vi "XY Graph Compute Convolution Product Event.vi"(6 "Reference Decay":T1, 8 "Error In":errorcluster, 9 "Valid Reference Decay?":bool, 10 "Plot at Coordinates":i32, 11 "Multiplot XY Graph":T2) -> (0 "Error Out":errorcluster, 1 "Message":string, 3 "Plot Name":string)   [LabVIEW 2021, in "XY Graph Add-Ons.lvlib"]
uses:
  XY Graph Add-Ons.lvlib
  XY Graph Refnum.ctl
  XY Plot Data.ctl
  Fits/Fits.lvlib
  Math/Math.lvlib
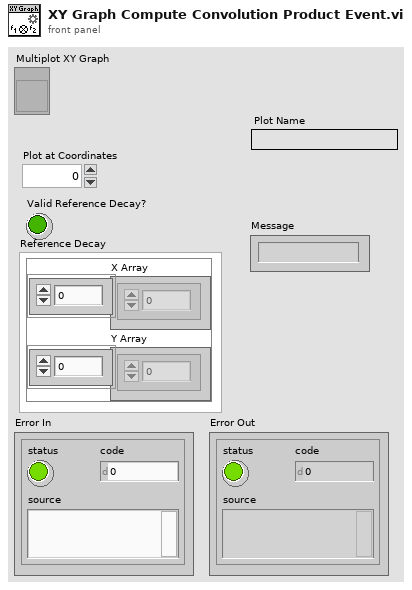
[diagram p1: front panel]
types:
  T1 = typedef "XY Graph Add-Ons.lvlib/XY Plot Data.ctl" = cluster{"X Array":dbl[], "Y Array":dbl[]}
  T2 = typedef "XY Graph Add-Ons.lvlib/XY Graph Refnum.ctl" = refnum<vi>
  T3 = typedef "Graphs.lvlib/Plot Destination.ctl" = enum32{"Plot 1", "Plot 2", "New Plot"}
  T4 = typedef "XY Graph Add-Ons.lvlib/XY Graph Convolution Product Options.ctl" = cluster{"Plot 1":u16, "Plot 2":u16, "Period Type":T5, "Period":dbl[unit], "Time Step":T6, "Step":dbl[unit]}
  T5 = typedef "XY Graph Add-Ons.lvlib/XY Graph Convolution Period Type.ctl" = enum16{"Laser", "Plot 1 Duration", "Plot 2 Duration", "User Defined"}
  T6 = typedef "XY Graph Add-Ons.lvlib/XY Graph Convolution Step Type.ctl" = enum16{"Plot 1 Step", "Plot 2 Step", "User Defined"}
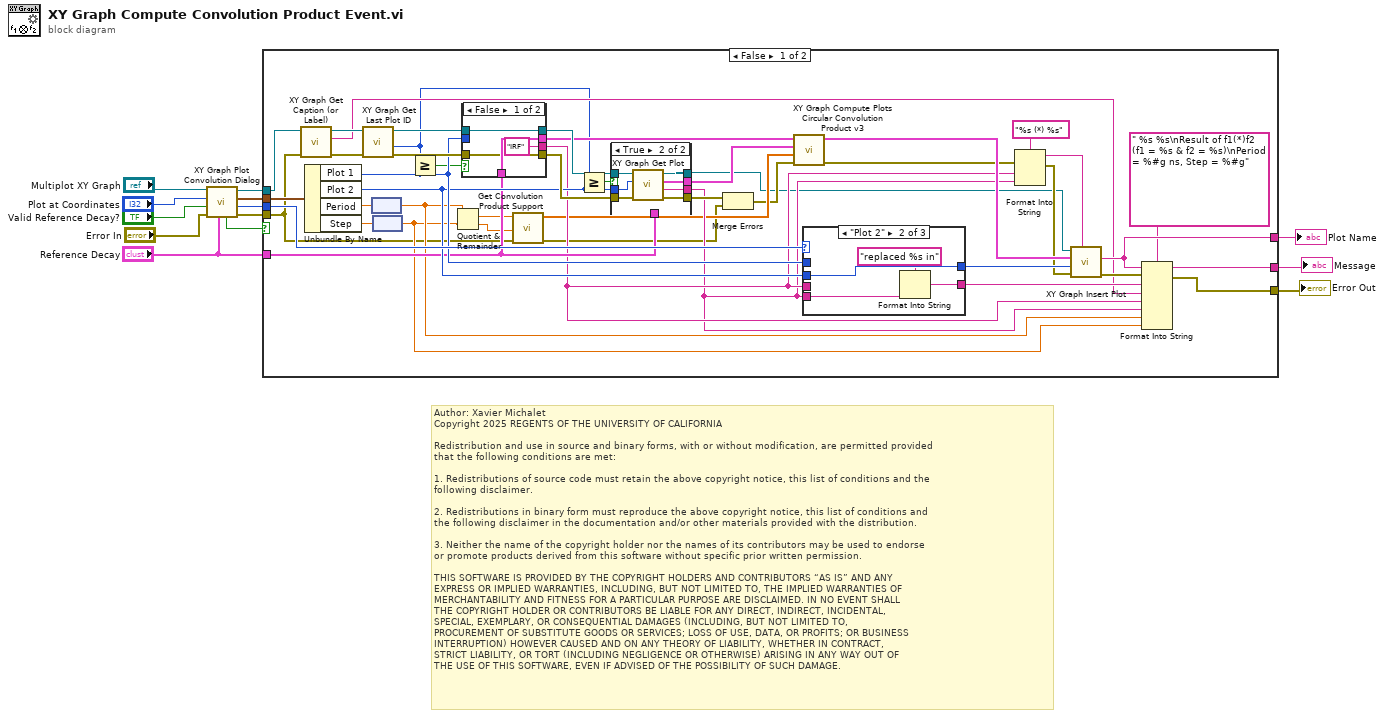
[diagram p0: block diagram]
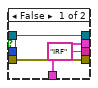
[diagram p2: hidden frame]
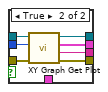
[diagram p3: hidden frame]
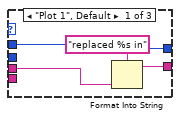
[diagram p4: hidden frame]
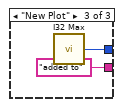
[diagram p5: hidden frame]
diagram:
  # "Author: Xavier Michalet\nCopyright 2025 REGENTS OF THE UNIVERSITY OF CALIFORNIA\n\nRedistribution and use in source and binary forms, with or without modification, are permitted provided\nthat the following conditions are met:\n\n1. Redistributions of source code must retain the above copyright notice, this list of conditions and the\nfollowing disclaimer.\n\n2. Redistributions in binary form must reproduce the above copyright notice, this list of conditions and\nthe following disclaimer in the documentation and/or other materials provided with the distribution.\n\n3. Neither the name of the copyright holder nor the names of its contributors may be used to endorse \nor promote products derived from this software without specific prior written permission.\n\nTHIS SOFTWARE IS PROVIDED BY THE COPYRIGHT HOLDERS AND CONTRIBUTORS “AS IS” AND ANY \nEXPRESS OR IMPLIED WARRANTIES, INCLUDING, BUT NOT LIMITED TO, THE IMPLIED WARRANTIES OF\nMERCHANTABILITY AND FITNESS FOR A PARTICULAR PURPOSE ARE DISCLAIMED. IN NO EVENT SHALL\nTHE COPYRIGHT HOLDER OR CONTRIBUTORS BE LIABLE FOR ANY DIRECT, INDIRECT, INCIDENTAL, \nSPECIAL, EXEMPLARY, OR CONSEQUENTIAL DAMAGES (INCLUDING, BUT NOT LIMITED TO, \nPROCUREMENT OF SUBSTITUTE GOODS OR SERVICES; LOSS OF USE, DATA, OR PROFITS; OR BUSINESS\nINTERRUPTION) HOWEVER CAUSED AND ON ANY THEORY OF LIABILITY, WHETHER IN CONTRACT, \nSTRICT LIABILITY, OR TORT (INCLUDING NEGLIGENCE OR OTHERWISE) ARISING IN ANY WAY OUT OF\nTHE USE OF THIS SOFTWARE, EVEN IF ADVISED OF THE POSSIBILITY OF SUCH DAMAGE."
  n1 = call "XY Graph Plot Convolution Dialog.vi"("Reference Decay"="Reference Decay", "Error In"="Error In", "Valid Reference Decay?"="Valid Reference Decay?", "Plot at Coordinates"="Plot at Coordinates", "XY Graph"="Multiplot XY Graph") -> ("Error Out"=w6:errorcluster, "Plot Destination out"=w4:T3, "Convolution Product Options out"=w3:T4, "XY Graph (dup)"=w2:refnum<vi>, "Cancelled"=w5:bool)  [unwired: 2 in]
  n2 = case shown="False" w5 {
    tunnel: [w56 w89] -> w13
    tunnel: [w55 _] -> w12
    tunnel: [w54 _] -> w11
    tunnel: w6 -> [w17 w89]
    tunnel: w4 -> [w53 _]
    tunnel: w3 -> [w52 _]
    tunnel: w2 -> [w44 _]
    tunnel: "Reference Decay" -> [w28 _]
    frame False {
      n3 = call "XY Graph Get Caption (or Label).vi"("error in (no error)"=w17, "XYGraph in"=w44) -> ("error out"=w34:errorcluster, "Caption (or Label) Text"=w33:string, "XYGraph out"=w35:T2)  [unwired: 7 in]
      n4 = Unbundle By Name(w52) -> ("Plot 1"=w36:u16, "Plot 2"=w31:u16, "Period"=w47:dbl[unit], "Step"=w46:dbl[unit])
      n5 = call "XY Graph Get Last Plot ID.vi"("error in (no error)"=w34, "XYGraph in"=w35) -> ("error out"=w37:errorcluster, "Last Plot ID"=w30:i32, "XYGraph out"=w38:refnum<vi>)  [unwired: 7 in]
      n6 = node(w47) -> (w21:dbl)
      n7 = node(w46) -> (w20:dbl)
      n8 = Greater Or Equal?(x=w30, y=w36) -> (x >= y?=w32:bool)
      n9 = Quotient & Remainder(x=w21, y=w20) -> (floor(x/y)=w18:dbl)  [unwired: 1 out]
      n10 = case shown="False" w32 {
        tunnel: ["IRF" ("Plot Name") w78] -> w24
        tunnel: [w71 w77] -> w45
        tunnel: [w68 w76] -> w43
        tunnel: [w70 w75] -> w41
        tunnel: w38 -> [w71 w74]
        tunnel: w37 -> [w68 w73]
        tunnel: w36 -> [_ w72]
        tunnel: w28 -> [w70 _]
        frame False {
        }
        frame True {
          n11 = call "XY Graph Get Plot.vi"("error in (no error)"=w73, "Plot Index (-1: last)"=w72, "XYGraph in"=w74) -> ("error out"=w76:errorcluster, "Plot Name"=w78:string, "Plot Data"=w75:T1, "XYGraph out"=w77:T2)  [unwired: 4 in, 1 out]
        }
      }
      n12 = call "Get Convolution Product Support.vi"("Error In"=w17, "# Values"=w18, "IRF Period"=w21) -> ("Error Out"=w15:errorcluster, "Ramp"=w19:dbl[])  [unwired: 6 in, 1 out]
      n13 = Greater Or Equal?(x=w30, y=w31) -> (x >= y?=w29:bool)
      n14 = case shown="True" w29 {
        tunnel: [w60 w67] -> w14
        tunnel: ["IRF" ("Plot Name") w66] -> w23
        tunnel: w45 -> [w60 w65]
        tunnel: w43 -> [w58 w64]
        tunnel: w31 -> [_ w61]
        tunnel: [w58 w63] -> w42
        tunnel: [w59 w62] -> w40
        tunnel: w28 -> [w59 _]
        frame False {
        }
        frame True {
          n15 = call "XY Graph Get Plot.vi"("error in (no error)"=w64, "Plot Index (-1: last)"=w61, "XYGraph in"=w65) -> ("error out"=w63:errorcluster, "Plot Name"=w66:string, "Plot Data"=w62:T1, "XYGraph out"=w67:T2)  [unwired: 4 in, 1 out]
        }
      }
      n16 = Merge Errors(w42, w15) -> (w16:errorcluster)
      n17 = call "XY Graph Compute Plots Circular Convolution Product v3.vi"("Error In"=w16, "Support Axis (kernel's)"=w19, "Plot 2 (kernel)"=w40, "Plot 1 (function)"=w41) -> ("Error Out"=w27:errorcluster, "Convolution Product"=w39:T1)  [unwired: 5 in, 1 out]
      n18 = case shown="\"Plot 2\"" w53 {
        tunnel: w36 -> [w82 _ _]
        tunnel: [w82 w86 w87] -> w50
        tunnel: w31 -> [_ w86 _]
        tunnel: [w81 w85 "added to" ("input 1")] -> w48
        tunnel: w24 -> [w79 _ _]
        tunnel: w23 -> [_ w83 _]
        frame "Plot 1", Default {
          n19 = Format Into String(format string="replaced %s in" ("input 1"), w79) -> (resulting string=w81:string)  [unwired: 2 in, 1 out]
        }
        frame "Plot 2" {
          n20 = Format Into String(format string="replaced %s in" ("input 1"), w83) -> (resulting string=w85:string)  [unwired: 2 in, 1 out]
        }
        frame "New Plot" {
          n21 = call "I32 Max.vi"() -> ("I32 max"=w87:i32)
        }
      }
      n22 = Format Into String(format string="%s (*) %s", error in=w27, w24, w23) -> (resulting string=w22:string, error out=w26:errorcluster)  [unwired: 1 in]
      n23 = call "XY Graph Insert Plot.vi"("New Plot Name (Unchanged: \"\")"=w22, "Error In"=w26, "Plot Index (Default Inf: Append to End)"=w50, "New Plot"=w39, "Multiplot XY Graph Refnum in"=w14) -> ("Error Out"=w49:errorcluster, "Plot Name"=w54:string)  [unwired: 4 in, 1 out]
      n24 = Format Into String(format string=" %s %s\nResult of f1(*)f2 (f1 = %s & f2 = %s)\nPeriod = %#g ns, Step = %#g", initial string=w54, error in=w49, w48, w33, w24, w23, w21, w20) -> (resulting string=w55:string, error out=w56:errorcluster)
    }
    frame True {
      # "cancelled"
    }
  }
  "Error Out" <- w13
  "Message" <- w12
  "Plot Name" <- w11
